vi "Configure Session.vi"(8 "error in":errorcluster, 11 "Plugin in":refnum<class "Performanced XNET CAN Signal Logger.lvclass">) -> (0 "error out":errorcluster, 3 "Plugin out":refnum<class "Performanced XNET CAN Signal Logger.lvclass">)   [LabVIEW 2021, in "Performanced XNET CAN Signal Logger.lvlib" / "Performanced XNET CAN Signal Logger.lvclass"]
uses:
  Performanced XNET CAN Signal Logger.lvclass
  C:/Program Files/National Instruments/LabVIEW 2021/vi.lib/FlexLogger/SDK/PluginSDK.lvlibp/PEFClasses/SDK/Plugin/Plugin.lvclass
  <vilib>/FlexLogger/SDK/PluginSDK.lvlibp/PEFClasses/SDK/Plugin/ParameterAccess/Read Enum.vi
  <vilib>/FlexLogger/SDK/PluginSDK.lvlibp/PEFClasses/SDK/Plugin/ParameterAccess/Read DBL.vi
  <vilib>/FlexLogger/SDK/PluginSDK.lvlibp/PEFClasses/SDK/Plugin/Plugin.lvclass
  C:/Program Files/National Instruments/LabVIEW 2021/vi.lib/FlexLogger/SDK/PluginSDK.lvlibp/PEFClasses/SDK/Processing Element/Processing Element.lvclass
  C:/Users/NI/Desktop/NIO DongZulong FlexLogger XNET/XNET-CAN-Signal-Logger/src/FlexLogger Plugin/Performanced XNET CAN Signal Logger.lvclass
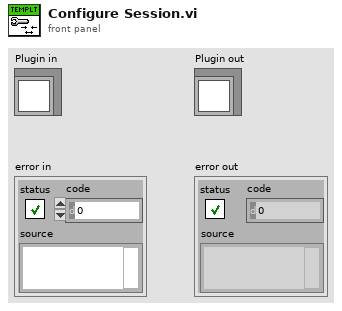
[diagram p1: front panel]
types:
  T1 = typedef "XNET-CAN-Signal-Logger.lvlib/Def-CAN Port Configuration.ctl" = cluster{"CAN Interface":refnum<k21>, "XNET Cluster":refnum<k21>, "#Signals":i32, "Sample Rate (Hz)":dbl}
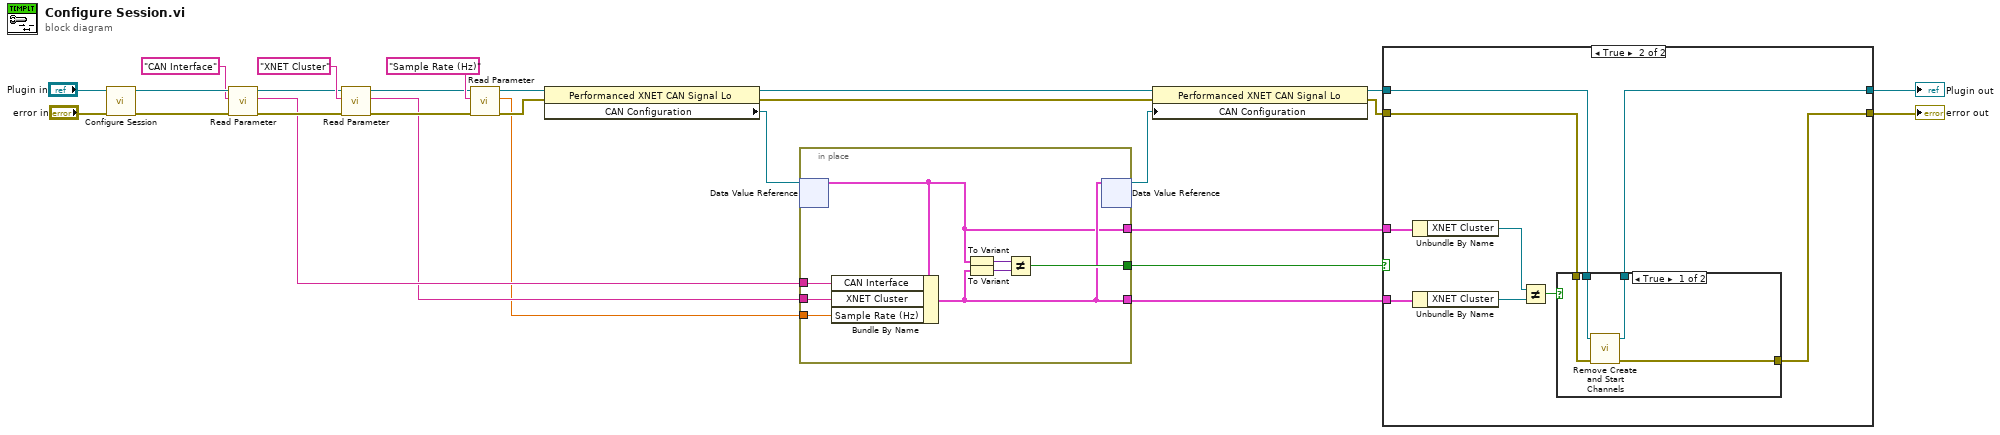
[diagram p0: block diagram]
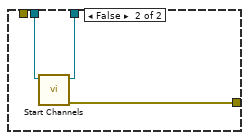
[diagram p3: hidden frame]
diagram:
  n1 = call-parent "Configure Session.vi"("error in (no error)"="error in", "Processing Element in"="Plugin in") -> ("error out"=w19:errorcluster, "Processing Element out"=w21:refnum<class "Performanced XNET CAN Signal Logger.lvclass">)  [unwired: 8 in]
  n2 = call-poly <vilib>:"Read Parameter.vi"("error in (no error)"=w19, "Name"="CAN Interface", "Plugin in"=w21) -> ("error out"=w16:errorcluster, "Value"=w10:string, "Plugin out"=w17:refnum<class "Performanced XNET CAN Signal Logger.lvclass">)  [unwired: 4 in, 2 out]
  n3 = call-poly <vilib>:"Read Parameter.vi"("error in (no error)"=w16, "Name"="XNET Cluster", "Plugin in"=w17) -> ("error out"=w13:errorcluster, "Value"=w9:string, "Plugin out"=w14:refnum<class "Performanced XNET CAN Signal Logger.lvclass">)  [unwired: 4 in, 2 out]
  n4 = call-poly <vilib>:"Read Parameter.vi"("error in (no error)"=w13, "Name"="Sample Rate (Hz)", "Plugin in"=w14) -> ("error out"=w11:errorcluster, "Value"=w8:dbl, "Plugin out"=w12:refnum<class "Performanced XNET CAN Signal Logger.lvclass">)  [unwired: 5 in, 1 out]
  n5 = property class="Performanced XNET CAN Signal Lo"(reference=w12, error in=w11) -> (reference out=w25:refnum<class "Performanced XNET CAN Signal Logger.lvclass">, error out=w3:errorcluster, "CAN Configuration"=w6:refnum<data-value>)
  n6 = in-place {
    in-place-border: [w33] -> w24
    in-place-border: w10 -> [w32]
    in-place-border: w9 -> [w31]
    in-place-border: w8 -> [w30]
    in-place-border: [w29] -> w7
    in-place-border: [w28] -> w5
    n7 = in-place-dvr #1(w6) -> (w28:T1)  [unwired: 1 out]
    n8 = Bundle By Name(cluster=w28, "CAN Interface"=w32, "XNET Cluster"=w31, "Sample Rate (Hz)"=w30) -> (w29:T1)
    n9 = To Variant(anything=w28) -> (Variant=w35:variant)
    n10 = To Variant(anything=w29) -> (Variant=w34:variant)
    n11 = Not Equal?(x=w35, y=w34) -> (x != y?=w33:bool)
    n12 = in-place-dvr #1(w29) -> (w1:refnum<data-value>)  [unwired: 1 out]
  }
  n13 = property class="Performanced XNET CAN Signal Lo"(reference=w25, error in=w3, "CAN Configuration"=w1) -> (reference out=w4:refnum<class "Performanced XNET CAN Signal Logger.lvclass">, error out=w2:errorcluster)
  n14 = case shown="True" w24 {
    tunnel: [w37 w43] -> w22
    tunnel: w4 -> [w37 w46]
    tunnel: [w36 w42] -> w23
    tunnel: w2 -> [w36 w44]
    tunnel: w7 -> [_ w41]
    tunnel: w5 -> [_ w39]
    frame False {
    }
    frame True {
      n15 = Unbundle By Name(w39) -> ("XNET Cluster"=w40:refnum<k21>)
      n16 = Unbundle By Name(w41) -> ("XNET Cluster"=w38:refnum<k21>)
      n17 = Not Equal?(x=w40, y=w38) -> (x != y?=w45:bool)
      n18 = case shown="True" w45 {
        tunnel: w46 -> [w50 w53]
        tunnel: [w49 w52] -> w43
        tunnel: [w48 w51] -> w42
        tunnel: w44 -> [w47 _]
        frame True {
          n19 = call-dynamic "Remove Create and Start Channels.vi"("error in (no error)"=w47, "Performanced XNET CAN Signal Logger in"=w50) -> ("error out"=w48:errorcluster, "Performanced XNET CAN Signal Logger out"=w49:refnum<class "Performanced XNET CAN Signal Logger.lvclass">)  [unwired: 8 in]
        }
        frame False {
          n20 = call-dynamic "Start Channels.vi"("Performanced XNET CAN Signal Logger in"=w53) -> ("error out"=w51:errorcluster, "Performanced XNET CAN Signal Logger out"=w52:refnum<class "Performanced XNET CAN Signal Logger.lvclass">)  [unwired: 9 in]
        }
      }
    }
  }
  "error out" <- w23
  "Plugin out" <- w22
